vi "DSF.Memory.BufferPool.Obtain Buffer.vi"(8 "error in (no error)":errorcluster, 9 "timeout ms (0)":i32 format="%d ms", 11 "BufferPool in":refnum<class "DSF.Memory.BufferPool.lvclass">) -> (0 "error out":errorcluster, 1 "timed out?":bool, 2 "Buffer":refnum<class "DSF.Memory.Buffer.lvclass">, 3 "BufferPool out":refnum<class "DSF.Memory.BufferPool.lvclass">)   [LabVIEW 2016, in "DSF.Memory.lvlib" / "DSF.Memory.BufferPool.lvclass"]
uses:
  DSF.Memory.BufferPool.lvclass
  Memory.Buffer/DSF.Memory.Buffer.lvclass
  DSF.Memory.BufferPool.lvclass/DSF.Memory.BufferPool.ctl
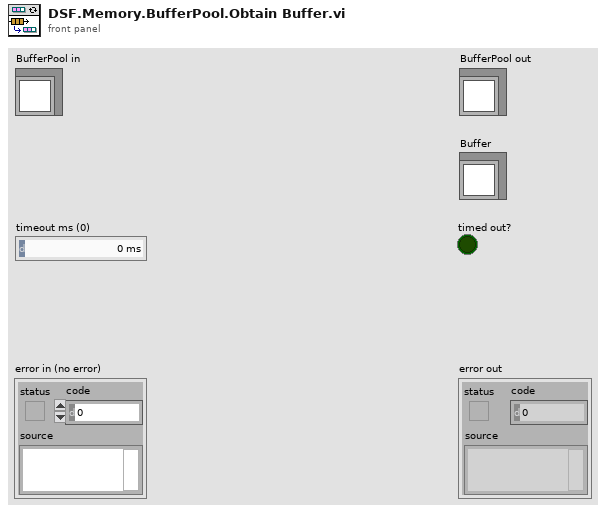
[diagram p1: front panel]
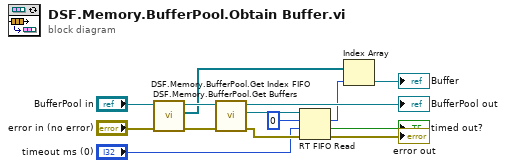
[diagram p0: block diagram]
diagram:
  n1 = call "DSF.Memory.BufferPool.Get Buffers.vi"("error in (no error)"="error in (no error)", "BufferPool in"="BufferPool in") -> ("error out"=w7:errorcluster, "Buffers"=w6:refnum<class "DSF.Memory.Buffer.lvclass">[], "BufferPool out"=w8:refnum<class "DSF.Memory.BufferPool.lvclass">)  [unwired: 7 in]
  n2 = call "DSF.Memory.BufferPool.Get Index FIFO.vi"("error in (no error)"=w7, "BufferPool in"=w8) -> ("error out"=w13:errorcluster, "Index FIFO"=w14:refnum<k33>, "BufferPool out"=→"BufferPool out":refnum<class "DSF.Memory.BufferPool.lvclass">)  [unwired: 7 in]
  n3 = RT FIFO Read(0:w14, 1:0, 2:"timeout ms (0)", 3:w13) -> (9:w3:i32, 10:→"timed out?":bool, 11:→"error out":errorcluster)  [unwired: 2 out]
  n4 = Index Array(array=w6, index=w3) -> (element=→"Buffer":refnum<class "DSF.Memory.Buffer.lvclass">)
